vi "Run.vi"(8 "error in (no error)":errorcluster, 11 "Audio Output Queue":refnum<queue>) -> (0 "error out":errorcluster)   [LabVIEW 2018, in "Audio Engine.lvlib"]
doc: "The main audio processing loop.\n\n<b>Priority:</b> Above Normal\n<b>Execution System:</b> Standard"
uses:
  Audio Engine/Audio Engine.lvlib
  Audio Output/Audio Output Queue Type.ctl
  Classes/Deck/Deck.lvclass
  Classes/Mixer/Mixer.lvclass
  Audio Output/Audio Output.lvlib
  Audio Processing.lvlib
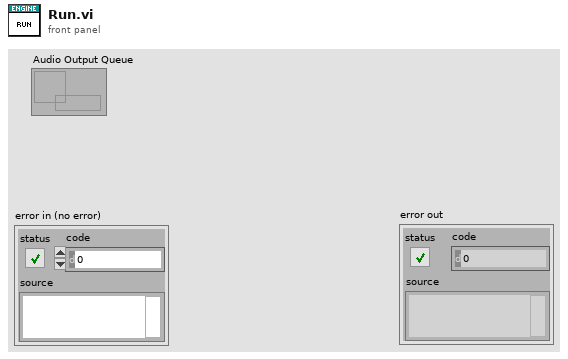
[diagram p1: front panel]
types:
  T1 = typedef "Audio Output.lvlib/Audio Output Queue Type.ctl" = cluster{"Master":waveform(i16)[], "Headphones":waveform(i16)[]}
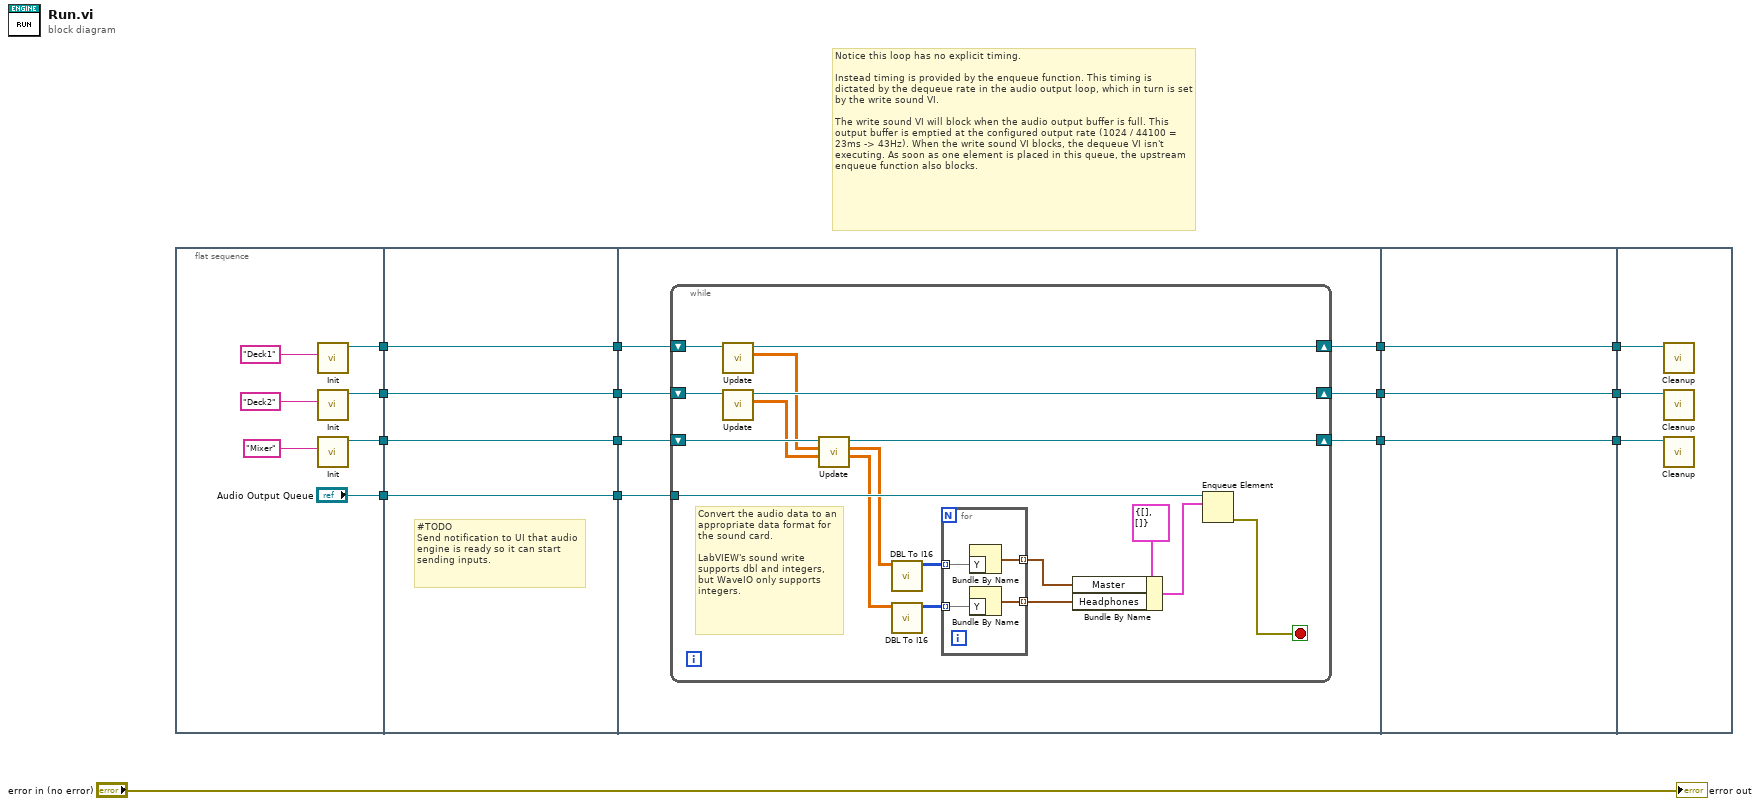
[diagram p0: block diagram]
diagram:
  # "Notice this loop has no explicit timing. \n\nInstead timing is provided by the enqueue function. This timing is dictated by the dequeue rate in the audio output loop, which in turn is set by the write sound VI.\n\nThe write sound VI will block when the audio output buffer is full. This output buffer is emptied at the configured output rate (1024 / 44100 = 23ms -> 43Hz). When the write sound VI blocks, the dequeue VI isn't executing. As soon as one element is placed in this queue, the upstream enqueue function also blocks."
  n1 = flat-sequence {
    tunnel: ["Audio Output Queue"] -> w14
    tunnel: [w18] -> w13
    tunnel: [w17] -> w12
    tunnel: [w16] -> w11
    tunnel: w14 -> [w26]
    tunnel: w13 -> [w25]
    tunnel: w12 -> [w24]
    tunnel: w11 -> [w23]
    tunnel: [w26] -> w10
    tunnel: [w25] -> w9
    tunnel: [w24] -> w8
    tunnel: [w23] -> w7
    tunnel: w10 -> [w33]
    tunnel: w9 -> [w27]
    tunnel: w8 -> [w28]
    tunnel: w7 -> [w29]
    tunnel: [w32] -> w5
    tunnel: [w31] -> w3
    tunnel: [w30] -> w1
    tunnel: [w58] -> w6
    tunnel: w5 -> [w58]
    tunnel: [w57] -> w4
    tunnel: w3 -> [w57]
    tunnel: [w56] -> w2
    tunnel: w1 -> [w56]
    tunnel: w6 -> [w61]
    tunnel: w4 -> [w60]
    tunnel: w2 -> [w59]
    frame #0 {
      n2 = call "Init.vi"("ID"="Deck1") -> ("Deck out"=w18:refnum<class "Deck.lvclass">)  [unwired: 9 in, 1 out]
      n3 = call "Init.vi"("ID"="Deck2") -> ("Deck out"=w17:refnum<class "Deck.lvclass">)  [unwired: 9 in, 1 out]
      n4 = call "Init.vi"("ID"="Mixer") -> ("Mixer out"=w16:refnum<class "Mixer.lvclass">)  [unwired: 9 in, 1 out]
    }
    frame #1 {
      # "#TODO\nSend notification to UI that audio engine is ready so it can start sending inputs."
    }
    frame #2 {
      n5 = while {
        shift-right: [w50] -> w32
        shift-left: w27 -> [w51]
        tunnel: w33 -> [w49]
        shift-right: [w46] -> w31
        shift-left: w28 -> [w47]
        shift-right: [w44] -> w30
        shift-left: w29 -> [w45]
        stop <- w48 stop-if-true
        # "Convert the audio data to an appropriate data format for the sound card.\n\nLabVIEW's sound write supports dbl and integers, but WaveIO only supports integers."
        n6 = call "Update.vi"("Deck in"=w51) -> ("Audio Block"=w43:dbl[][], "Deck out"=w50:refnum<class "Deck.lvclass">)  [unwired: 8 in, 1 out]
        n7 = call "Update.vi"("Deck in"=w47) -> ("Audio Block"=w42:dbl[][], "Deck out"=w46:refnum<class "Deck.lvclass">)  [unwired: 8 in, 1 out]
        n8 = call "Update.vi"("Audio Block 2"=w42, "Audio Block 1"=w43, "Mixer in"=w45) -> ("Headphones Audio Block Out"=w35:dbl[][], "Master Audio Block Out"=w37:dbl[][], "Mixer out"=w44:refnum<class "Mixer.lvclass">)  [unwired: 5 in, 1 out]
        n9 = call "DBL To I16.vi"("Audio Data (2D DBL)"=w37) -> ("Audio Data (2D I16)"=w36:i16[][])  [unwired: 9 in, 1 out]
        n10 = call "DBL To I16.vi"("Audio Data (2D DBL)"=w35) -> ("Audio Data (2D I16)"=w34:i16[][])  [unwired: 9 in, 1 out]
        n11 = for {
          tunnel: w36 -> [w55] mode=indexing
          tunnel: [w54] -> w40 mode=indexing
          tunnel: w34 -> [w53] mode=indexing
          tunnel: [w52] -> w39 mode=indexing
          n12 = Bundle By Name("Y"=w55) -> (w54:waveform(i16))  [unwired: 1 in]
          n13 = Bundle By Name("Y"=w53) -> (w52:waveform(i16))  [unwired: 1 in]
        }
        n14 = Bundle By Name(cluster=T1 {"Master"=[], "Headphones"=[]}, "Master"=w40, "Headphones"=w39) -> (w38:T1)
        n15 = Enqueue Element(queue=w49, element=w38) -> (error out=w48:errorcluster)  [unwired: 2 in, 2 out]
      }
    }
    frame #3 {
    }
    frame #4 {
      n16 = call "Cleanup.vi"("Deck in"=w61) -> ()  [unwired: 9 in, 2 out]
      n17 = call "Cleanup.vi"("Deck in"=w60) -> ()  [unwired: 9 in, 2 out]
      n18 = call "Cleanup.vi"("Mixer in"=w59) -> ()  [unwired: 9 in, 2 out]
    }
  }
  "error out" <- "error in (no error)"
